vi "Select Threat Details.vi"(2 "threatGroup":string) -> (0 "threatDetails":string[](array[string]))   [LabVIEW 2015]
panel:
  out "error OUT":errorcluster
  in  "error IN":errorcluster
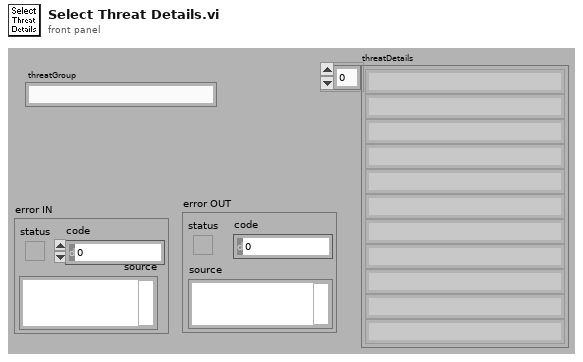
[diagram p1: front panel]
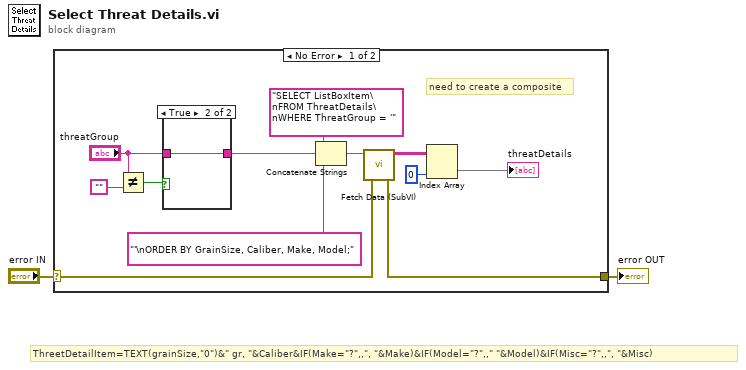
[diagram p0: block diagram]
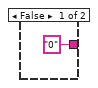
[diagram p2: hidden frame]
diagram:
  # "ThreetDetailItem=TEXT(grainSize,\"0\")&\" gr, \"&Caliber&IF(Make=\"?\",,\", \"&Make)&IF(Model=\"?\",,\" \"&Model)&IF(Misc=\"?\",,\", \"&Misc)"
  n1 = case shown="No Error" "error IN" {
    selector: "error IN" -> [w5 w17]
    tunnel: [w4 w17] -> w1
    frame No Error {
      # "need to create a composite"
      n2 = Not Equal?(x="threatGroup", y="") -> (x != y?=w8:bool)
      n3 = case shown="True" w8 {
        tunnel: ["0" ("projectileWeight") w16] -> w6
        tunnel: "threatGroup" -> [_ w16]
        frame False {
        }
        frame True {
        }
      }
      n4 = Concatenate Strings("SELECT ListBoxItem\nFROM ThreatDetails\nWHERE ThreatGroup = '", w6, "'\nORDER BY GrainSize, Caliber, Make, Model;" ("string")) -> (w10:string)
      n5 = call "Fetch Data (SubVI).vi"("error IN"=w5, "query string"=w10) -> ("error OUT"=w4:errorcluster, "recordset data"=w14:string[][])  [unwired: 4 out]
      n6 = Index Array(array=w14, index (col)=0 ("disabled index (col)")) -> (element=→"threatDetails":string[])  [unwired: 1 in]
    }
    frame Error {
    }
  }
  "error OUT" <- w1
